vi "Keithley2100subVI_V2.vi"(11 "K-2100 init":T1) -> (1 "String":string, 2 "Measurement":dbl, 3 "Cluster":T1)   [LabVIEW 2014]
uses:
  Drivers and Software/Keithley 2100 Series/Keithley 2100 Series.lvlib
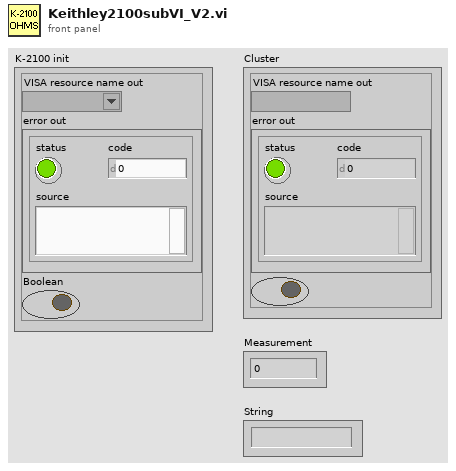
[diagram p1: front panel]
types:
  T1 = cluster{"VISA resource name out":refnum<visa-resource-name>, "error out":errorcluster, "Boolean":bool}
  T2 = cluster{"VISA resource name out":refnum<visa-resource-name>, "error out":errorcluster, bool}
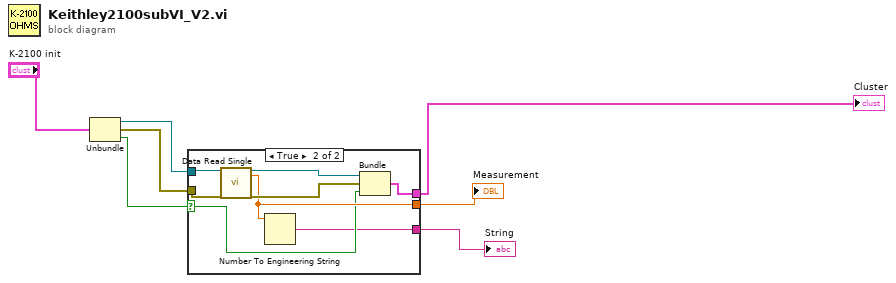
[diagram p0: block diagram]
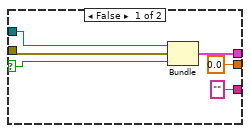
[diagram p2: hidden frame]
diagram:
  n1 = Unbundle("K-2100 init") -> ("VISA resource name out"=w4:refnum<visa-resource-name>, "error out"=w3:errorcluster, "Boolean"=w2:bool)
  n2 = case shown="True" w2 {
    selector: w2 -> [w11 w16]
    tunnel: w3 -> [w12 w21]
    tunnel: w4 -> [w13 w20]
    tunnel: [0.0 ("Measurement") w17] -> w5
    tunnel: [w10 w14] -> w7
    tunnel: ["" w15] -> w6
    frame False {
      n3 = Bundle("VISA resource name out"=w13, "error out"=w12, w11) -> (w10:T2)  [unwired: 1 in]
    }
    frame True {
      n4 = call "Data Read Single.vi"("VISA resource name"=w20, "error in (no error)"=w21) -> ("VISA resource name out"=w19:refnum<visa-resource-name>, "Measurement"=w17:dbl, "error out"=w18:errorcluster)  [unwired: 15 in]
      n5 = Number To Engineering String ("elapsed time (min)")(4:w17) -> (0:w15:string)  [unwired: 3 in]
      n6 = Bundle("VISA resource name out"=w19, "error out"=w18, w16) -> (w14:T2)  [unwired: 1 in]
    }
  }
  "Cluster" <- w7
  "String" <- w6
  "Measurement" <- w5
